vi "Configure Gain Phase Measurement.vi"(7 "Attenuation (20)":dbl=20.0, 8 "error in (no error)":errorcluster, 9 "Impedance (50)":dbl=50.0, 10 "Port (0: T)":i32(ring) items=["T Port", "R Port"], 11 "VISA resource name":refnum<visa-resource-name>) -> (0 "error out":errorcluster, 3 "VISA resource name out":refnum<visa-resource-name>)   [LabVIEW 2020, in "Agilent ENA Series.lvlib"]
doc: "Configures the gain phase measurement settings for T and R port.\n\n<B>Note:</B> This VI is only valid for E5061B."
uses:
  <instrlib>/Agilent ENA Series/Agilent ENA Series.lvlib
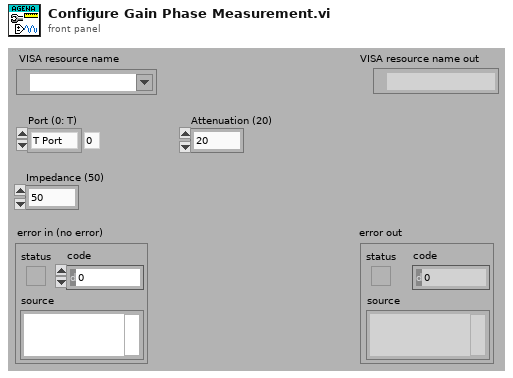
[diagram p1: front panel]
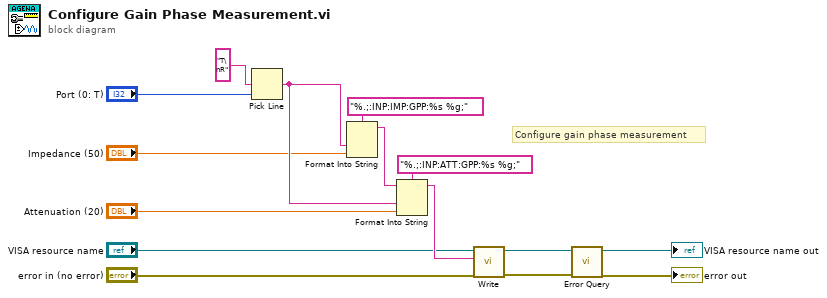
[diagram p0: block diagram]
diagram:
  # "Configure gain phase measurement"
  n1 = Pick Line(multi-line string="T\nR", line index="Port (0: T)") -> (output string=w12:string)  [unwired: 1 out]
  n2 = Format Into String(format string="%.;:INP:IMP:GPP:%s %g;", w12, "Impedance (50)") -> (resulting string=w6:string)  [unwired: 2 in, 1 out]
  n3 = Format Into String(format string="%.;:INP:ATT:GPP:%s %g;", initial string=w6, w12, "Attenuation (20)") -> (resulting string=w4:string)  [unwired: 1 in, 1 out]
  n4 = call <instrlib>:"Write.vi"("error in (no error)"="error in (no error)", "String ()"=w4, "VISA resource name"="VISA resource name") -> ("error out"=w1:errorcluster, "VISA resource name out"=w5:refnum<visa-resource-name>)  [unwired: 6 in, 1 out]
  n5 = call <instrlib>:"Error Query.vi"("error in (no error)"=w1, "VISA resource name"=w5) -> ("error out"=→"error out":errorcluster, "VISA resource name out"=→"VISA resource name out":refnum<visa-resource-name>)  [unwired: 8 out]
